vi "StoreFrameInfo.vi"(9 "frame":i32, 10 "ResultManager":T1, 11 "Timestamp":dbl) -> ()   [LabVIEW 2011]
uses:
  qtrk/QTrk.llb/ResultManagerInstance.ctl
  GlobalVariables.vi
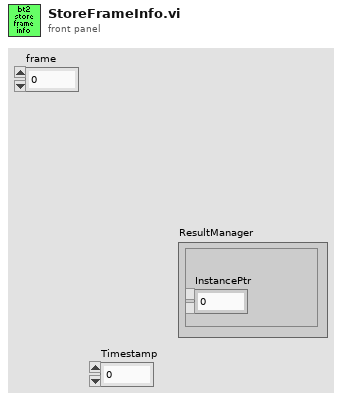
[diagram p1: front panel]
types:
  T1 = typedef "ResultManagerInstance.ctl" = cluster{"InstancePtr":u64}
  T2 = typedef "MotorStateType.ctl" = cluster{"Enabled?":bool, "Current Position":T3, "Update counter":i32}
  T3 = typedef "MotorPosType.ctl" = cluster{"Magnet Z":dbl, "Magnet rotation":dbl, "Camera":T4, "Piezo XY":T4, "Piezo Z":dbl}
  T4 = typedef "XYf.ctl" = cluster{"X":sgl, "Y":sgl}
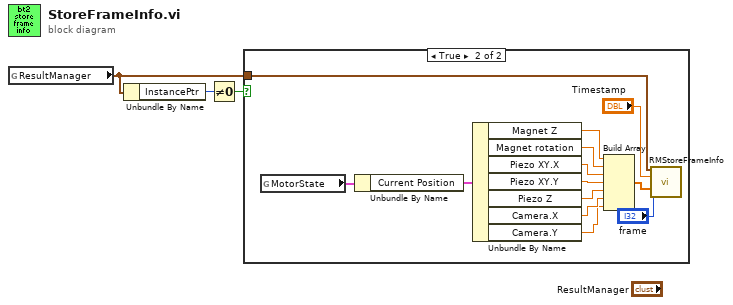
[diagram p0: block diagram]
diagram:
  n1 = global read "GlobalVariables.vi" "ResultManager"() -> (w3:T1)
  n2 = Unbundle By Name(w3) -> ("InstancePtr"=w1:u64)
  n3 = Not Equal To 0?(x=w1) -> (x != 0?=w2:bool)
  n4 = case shown="True" w2 {
    tunnel: w3 -> [_ w8]
    frame False {
    }
    frame True {
      n5 = global read "GlobalVariables.vi" "MotorState"() -> (w16:T2)
      n6 = Unbundle By Name(w16) -> ("Current Position"=w14:T3)
      n7 = Unbundle By Name(w14) -> ("Magnet Z"=w13:dbl, "Magnet rotation"=w12:dbl, "Piezo XY.X"=w11:sgl, "Piezo XY.Y"=w10:sgl, "Piezo Z"=w7:dbl, "Camera.X"=w6:sgl, "Camera.Y"=w5:sgl)
      n8 = Build Array(w13, w12, w11, w10, w7, w6, w5) -> (w9:dbl[])
      n9 = call "RMStoreFrameInfo.vi"("ResultManager"=w8, "timestamp"="Timestamp", "frame"="frame", "columns"=w9) -> ()  [unwired: 10 in, 2 out]
    }
  }
